vi "concatenated_string.vi"() -> ()   [LabVIEW 2019]
panel:
  out "resulting string 2":string
  in  "stop":bool
  out "resulting string":string
  out "value":dbl
  in  "Şehir":string
  in  "soyadi":string
  in  "adi":string
  out "concatenated string":string
  out "length":i32
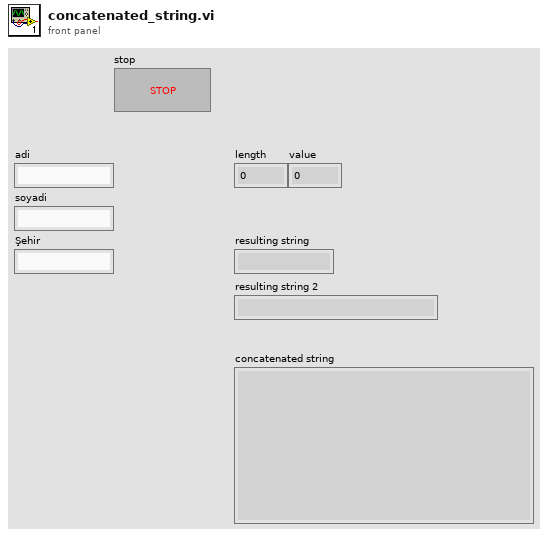
[diagram p1: front panel]
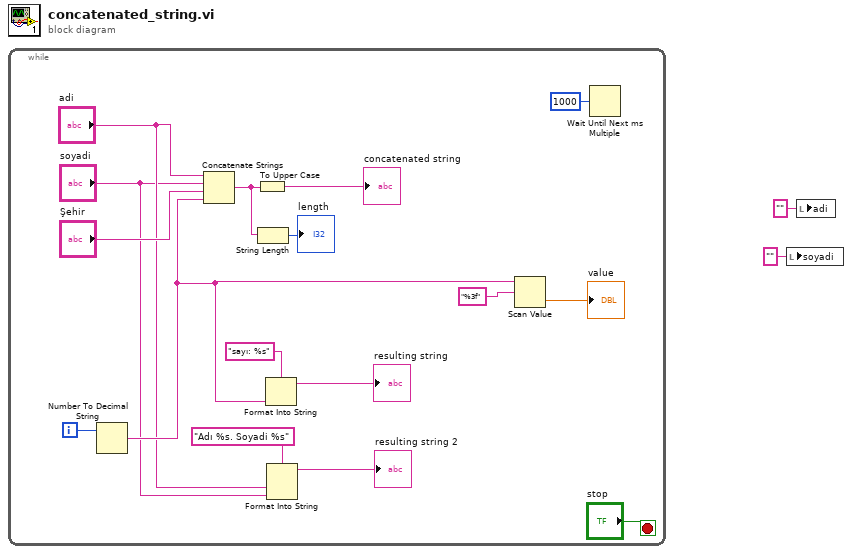
[diagram p0: block diagram]
diagram:
  n1 = while {
    i -> [w15]
    stop <- "stop" stop-if-true
    n2 = Number To Decimal String(number=w15) -> (decimal integer string=w9:string)  [unwired: 1 in]
    n3 = Concatenate Strings("adi", "soyadi", "Şehir", w9) -> (w14:string)
    n4 = To Upper Case(1:w14) -> (0:→"concatenated string":string)
    n5 = String Length(string=w14) -> (length=→"length":i32)
    n6 = Format Into String(format string="sayı: %s", w9) -> (resulting string=→"resulting string":string)  [unwired: 2 in, 1 out]
    n7 = Format Into String(format string="Adı %s. Soyadi %s", "adi", "soyadi") -> (resulting string=→"resulting string 2":string)  [unwired: 2 in, 1 out]
    n8 = Scan Value(string=w9, format string="%3f") -> (value=→"value":dbl)  [unwired: 1 in, 1 out]
    n9 = Wait Until Next ms Multiple(millisecond multiple=u32 1000) -> ()  [unwired: 1 out]
  }
  n10 = local write "soyadi"("" ("soyadi")) -> ()
  n11 = local write "adi"("" ("adi")) -> ()
